vi "加密与伪装.vi"() -> ()   [LabVIEW 2009]
panel:
  in  "解密":bool
  in  "伪装":bool
  in  "选取需要加密的文件夹":path
  # "文件夹加密工具"
  # "愤怒的企鹅  lucifer"
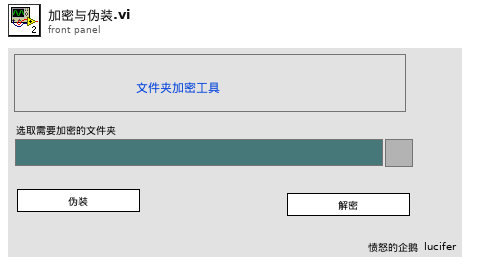
[diagram p1: front panel]
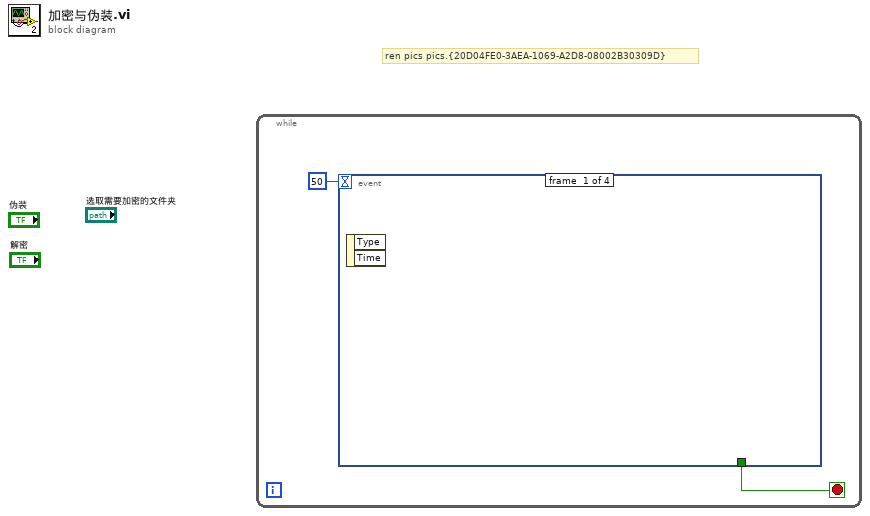
[diagram p0: block diagram]
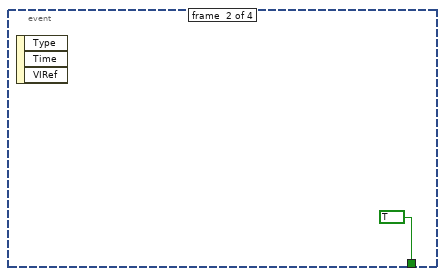
[diagram p2: hidden frame]
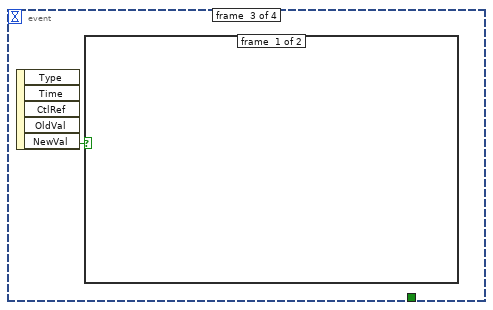
[diagram p3: hidden frame]
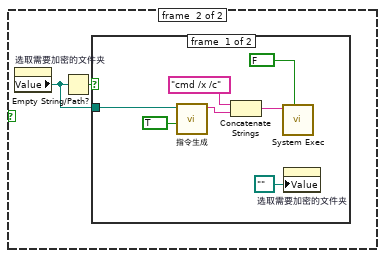
[diagram p4: hidden frame]
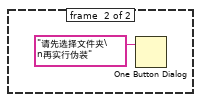
[diagram p5: hidden frame]
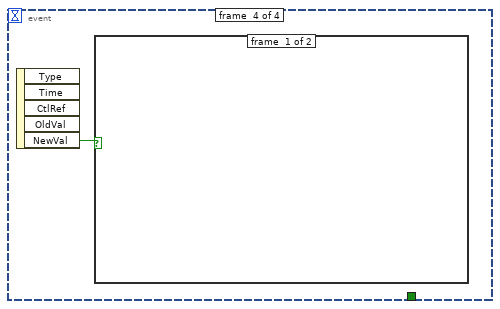
[diagram p6: hidden frame]
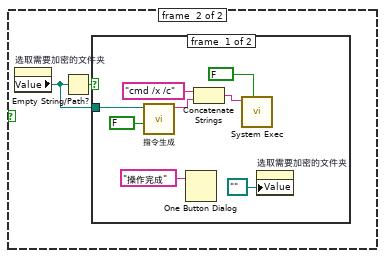
[diagram p7: hidden frame]
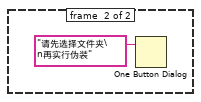
[diagram p8: hidden frame]
diagram:
  # "ren pics pics.{20D04FE0-3AEA-1069-A2D8-08002B30309D}"
  n1 = while {
    stop <- w1 stop-if-true
    n2 = event shown="[2] \"伪装\": 值改变" {
      selector: _ -> [_ _ _ _]
      dyn-events: _ -> [_ _ _ _]
      timeout: 50 -> [_ _ _ _]
      tunnel: [_ TRUE _ _] -> w1
      event #0 {
        n3 = event-data() -> ()  [unwired: 1 in, 2 out]
      }
      event #1 {
        n4 = event-data() -> ()  [unwired: 1 in, 3 out]
      }
      event #2 {
        n5 = event-data() -> ("NewVal"=w4:bool)  [unwired: 1 in, 4 out]
        n6 = case shown="真" w4 {
          frame #0 {
          }
          frame #1 {
            n7 = property on="选取需要加密的文件夹" class="Path"() -> ("Value"=w5:path)  [unwired: 2 in, 2 out]
            n8 = Empty String/Path?(string/path=w5) -> (empty?=w6:bool)
            n9 = case shown="假" w6 {
              tunnel: w5 -> [w12 _]
              frame #0 {
                n10 = call "指令生成.vi"("伪装\\解密"=TRUE ("伪装\\解密"), "路径"=w12) -> ("指令"=w9:string)  [unwired: 9 in]
                n11 = Concatenate Strings("cmd /x /c" ("字符串"), w9) -> (w8:string)
                n12 = call <vilib>:"System Exec.vi"("wait until completion? (T)"=FALSE, "command line"=w8) -> ()  [unwired: 6 in, 4 out]
                n13 = property on="选取需要加密的文件夹" class="Path"("Value"=path "" ("选取需要加密的文件夹")) -> ()  [unwired: 2 in, 2 out]
              }
              frame #1 {
                n14 = One Button Dialog(message="请先选择文件夹\n再实行伪装" ("消息")) -> ()  [unwired: 1 in, 1 out]
              }
            }
          }
        }
      }
      event #3 {
        n15 = event-data() -> ("NewVal"=w15:bool)  [unwired: 1 in, 4 out]
        n16 = case shown="真" w15 {
          frame #0 {
          }
          frame #1 {
            n17 = property on="选取需要加密的文件夹" class="Path"() -> ("Value"=w16:path)  [unwired: 2 in, 2 out]
            n18 = Empty String/Path?(string/path=w16) -> (empty?=w17:bool)
            n19 = case shown="假" w17 {
              tunnel: w16 -> [w24 _]
              frame #0 {
                n20 = call "指令生成.vi"("伪装\\解密"=FALSE ("伪装\\解密"), "路径"=w24) -> ("指令"=w20:string)  [unwired: 9 in]
                n21 = One Button Dialog(message="操作完成" ("消息")) -> ()  [unwired: 1 in, 1 out]
                n22 = Concatenate Strings("cmd /x /c" ("字符串"), w20) -> (w21:string)
                n23 = call <vilib>:"System Exec.vi"("wait until completion? (T)"=FALSE, "command line"=w21) -> ()  [unwired: 6 in, 4 out]
                n24 = property on="选取需要加密的文件夹" class="Path"("Value"=path "" ("选取需要加密的文件夹")) -> ()  [unwired: 2 in, 2 out]
              }
              frame #1 {
                n25 = One Button Dialog(message="请先选择文件夹\n再实行伪装" ("消息")) -> ()  [unwired: 1 in, 1 out]
              }
            }
          }
        }
      }
    }
  }
